vi "loop_for.vi"() -> ()   [LabVIEW 2019]
panel:
  out "Numeric":i32
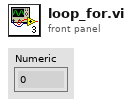
[diagram p1: front panel]
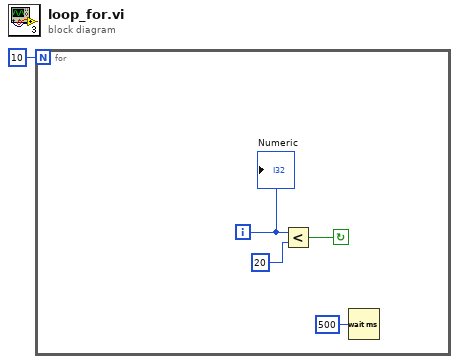
[diagram p0: block diagram]
diagram:
  n1 = for {
    N: 10 -> [_]
    i -> [w5]
    stop <- w3 continue-if-true
    n2 = Less?(x=w5, y=20) -> (x < y?=w3:bool)
    n3 = Wait (ms)(milliseconds to wait=u32 500) -> ()  [unwired: 1 out]
    "Numeric" <- w5
  }
